vi "GetImageRegistrations.vi"(8 "error in (no error)":errorcluster) -> (0 "error out":errorcluster, 2 "RegisterImage":T1[](array[typedef]))   [LabVIEW 2017, in "IrAcquisition.lvlib"]
uses:
  <vilib>/addons/InsightCM/Devices/Shared/Ir/IrAcquisition/IrAcquisition.lvlib
  <vilib>/addons/InsightCM/Devices/Shared/Ir/IrDataEventCreator/controls/RegisterImageRoutedMessage.ctl
  <vilib>/addons/InsightCM/Devices/Shared/Ir/IrDataEventCreator/controls/Registry_Image.ctl
  <vilib>/addons/InsightCM/MessageBus/Base/controls/KeyValuePair.ctl
  <vilib>/addons/InsightCM/Utilities/GlobalConfiguration/GlobalConfiguration.lvlib
  <vilib>/addons/InsightCM/Devices/Shared/Ir/IrDataEventCreator/IrDataEventCreator.lvlib
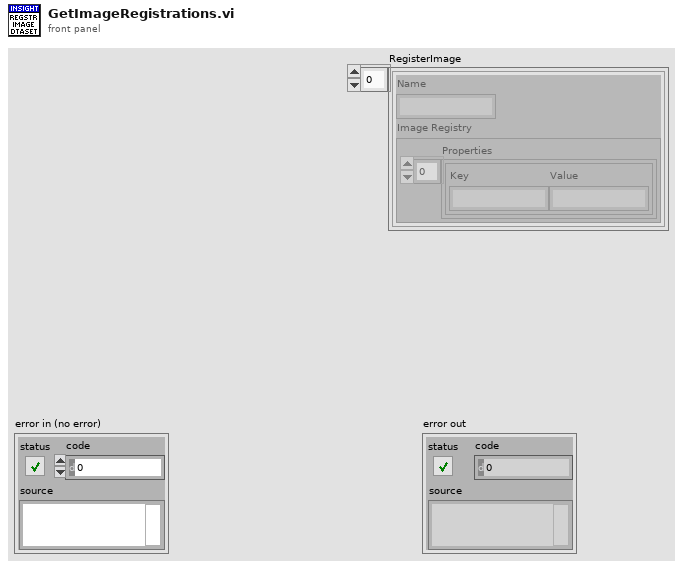
[diagram p1: front panel]
types:
  T1 = typedef "IrDataEventCreator.lvlib/RegisterImageRoutedMessage.ctl" = cluster{"Name":string, "Image Registry":T2}
  T2 = typedef "IrDataEventCreator.lvlib/Registry_Image.ctl" = cluster{"Properties":T3[]}
  T3 = typedef "KeyValuePair.ctl" = cluster{"Key":string, "Value":string}
  T4 = typedef "R2_DeviceModel.ctl" = cluster{"Device":T5, "Channels":T15[], "Tags":T17[]}
  T5 = typedef "R2_Device.ctl" = cluster{"Id":string, "Name":string, "DeviceType":string, "HardwareName":string, "IpAddress":string, "HardwareInfo":T3[], "ApplicationType":string, "ApplicationVersion":string, "EquipmentIds":string[], "ConfigurationVersion":string, "State":T6, "Properties":T3[], "DataGroups":T7[], "BurstModeTrigger":T11, "SensorGroups":T12[]}
  T6 = typedef "DeviceState.ctl" = cluster{"Disabled":bool}
  T7 = typedef "R2_DataGroup.ctl" = cluster{"Name":string, "OperatingStates":T8[], "Properties":T3[], "EquipmentIds":string[], "AssetNodeId":string}
  T8 = typedef "OperatingState.ctl" = cluster{"Name":string, "Properties":T3[], "Triggers":T9[]}
  T9 = typedef "Trigger.ctl" = cluster{"Type":string, "Expression":string, "Conditions":T10[]}
  T10 = typedef "Condition.ctl" = cluster{"Source":string, "Type":string, "Operator":string, "CompareTo":string, "DwellSeconds":dbl}
  T11 = typedef "BurstModeTrigger.ctl" = cluster{"Trigger":T9, "SampleRate":string, "AcquisitionLength":string}
  T12 = typedef "DeviceSensorGroup.ctl" = cluster{"EquipId":string, "SensorGroupId":string, "Endpoints":T13[]}
  T13 = typedef "Endpoint.ctl" = cluster{"Type":string, "Address":string, "Properties":T3[], "Channels":T14[]}
  T14 = typedef "WirelessChannel.ctl" = cluster{"ChannelNumber":i32, "AssetId":string}
  T15 = typedef "R2_Channel.ctl" = cluster{"Id":string, "DeviceId":string, "Name":string, "ChannelType":string, "HardwareKey":string, "HardwareChannel":string, "DataGroup":string, "Keywords":string[], "EquipmentIds":string[], "Properties":T3[], "Metrics":T16[], "AssetNodeId":string, "MeasType":string, "AssetName":string}
  T16 = typedef "Metric.ctl" = cluster{"Id":string, "Name":string, "Unit":string, "Properties":T3[], "MetricDefinitionInstanceId":string}
  T17 = typedef "Tag.ctl" = cluster{"Id":string, "Path":string, "Name":string, "Datatype":string, "Props":T3[], "Keywords":string[]}
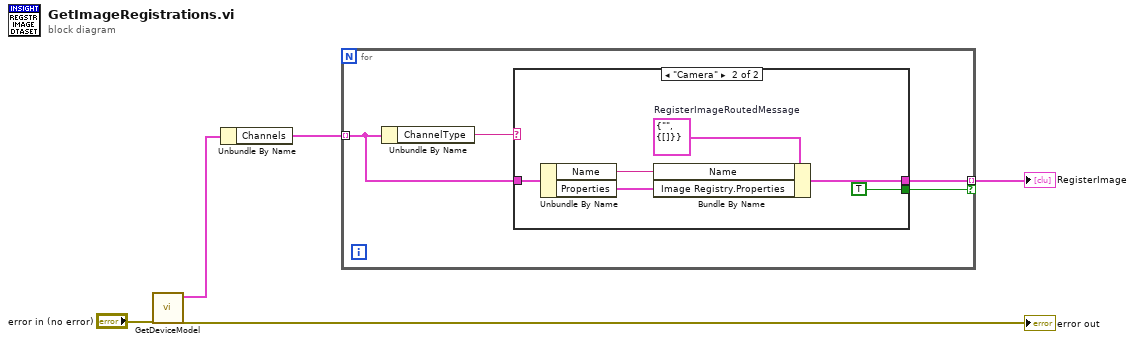
[diagram p0: block diagram]
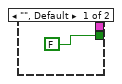
[diagram p2: hidden frame]
diagram:
  n1 = call <vilib>:"GetDeviceModel.vi"("error in (no error)"="error in (no error)") -> ("error out"=→"error out":errorcluster, "device model"=w4:T4)  [unwired: 8 in, 1 out]
  n2 = Unbundle By Name(w4) -> ("Channels"=w3:T15[])
  n3 = for {
    tunnel: w3 -> [w8] mode=indexing
    tunnel: [w7] -> w1 mode=indexing if=w6
    n4 = Unbundle By Name(w8) -> ("ChannelType"=w9:string)
    n5 = case shown="\"Camera\"" w9 {
      tunnel: w8 -> [_ w16]
      tunnel: [_ w14] -> w7
      tunnel: [FALSE TRUE] -> w6
      frame "", Default {
      }
      frame "Camera" {
        w11 = T1 {"Name"="", "Image Registry"={"Properties"=[]}}  # RegisterImageRoutedMessage
        n6 = Unbundle By Name(w16) -> ("Name"=w15:string, "Properties"=w12:T3[])
        n7 = Bundle By Name(cluster=w11, "Name"=w15, "Image Registry.Properties"=w12) -> (w14:T1)
      }
    }
  }
  "RegisterImage" <- w1
